vi "Execute Command.vi"(8 "error in (no error)":errorcluster, 9 "Command Name":string, 10 "Robot Actors.lvlib:Command.lvlib:Command.lvclass":refnum<class "Command.lvclass">, 11 "System Actor in":refnum<class "System Actor.lvclass">) -> (0 "error out":errorcluster, 3 "System Actor out":refnum<class "System Actor.lvclass">)   [LabVIEW 2013]
uses:
  <vilib>/ActorFramework/Actor/Actor.lvclass
  System Actor.lvclass
  Command/Command Class/Command.lvclass
  Command/Command Messages/Command Stopped Msg/Command Stopped Msg.lvclass
  Command/Command Messages/Command Started Msg/Command Started Msg.lvclass
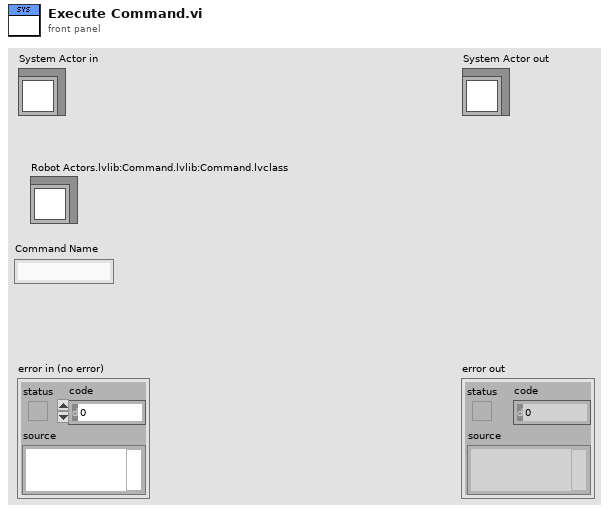
[diagram p1: front panel]
types:
  T1 = typedef "Robot Actors.lvlib/System Actor.lvlib/System Actor.lvclass/System Status.ctl" = cluster{"Instance Name":string, "Command Status":T2, "System Start Time":timestamp, "Next Command ID":dbl}
  T2 = typedef "Robot Actors.lvlib/Command.lvlib/Command.lvclass/Command Status.ctl" = cluster{"Command Name":string, "Command Start Time":timestamp, "Command End Time":timestamp, "Is Command Finished?":bool, "Command ID":dbl, "Command State":T3}
  T3 = typedef "Robot Actors.lvlib/Command.lvlib/Command.lvclass/Command States.ctl" = enum16{"Unknown", "Started", "Stopped", "Finished"}
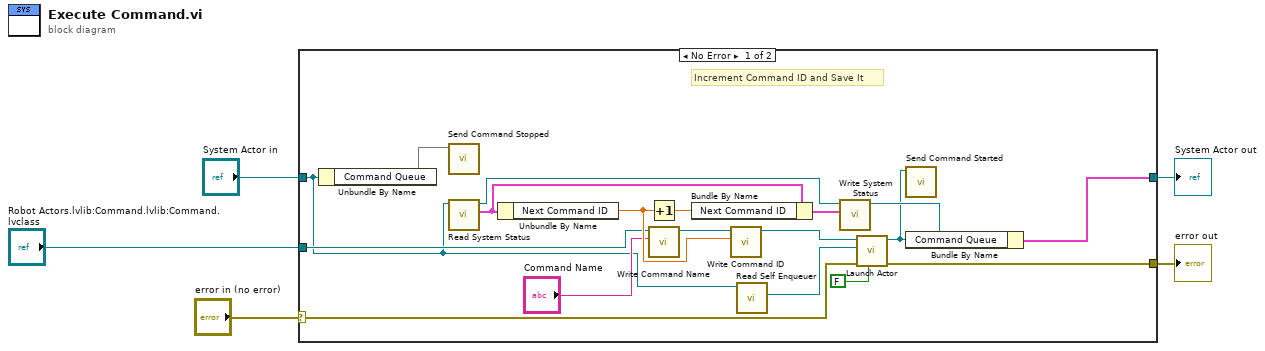
[diagram p0: block diagram]
diagram:
  n1 = case shown="No Error" "error in (no error)" {
    selector: "error in (no error)" -> [w21 w25]
    tunnel: [w22 w25] -> w4
    tunnel: [w20 w24] -> w2
    tunnel: "System Actor in" -> [w7 w24]
    tunnel: "Robot Actors.lvlib:Command.lvlib:Command.lvclass" -> [w10 _]
    frame No Error {
      # "Increment Command ID and Save It"
      n2 = Unbundle By Name(w7) -> ("Command Queue"=w8)
      n3 = call "Send Command Stopped.vi"("Message Enqueuer"=w8) -> ()  [unwired: 9 in, 2 out]
      n4 = call-dynamic "Read System Status.vi"("System Actor in"=w7) -> ("System Status"=w16:T1, "System Actor out"=w18:refnum<class "System Actor.lvclass">)  [unwired: 8 in, 1 out]
      n5 = Unbundle By Name(w16) -> ("Next Command ID"=w14:dbl)
      n6 = Increment(x=w14) -> (x+1=w13:dbl)
      n7 = call-dynamic "Write Command Name.vi"("Command Name"="Command Name", "Command in"=w10) -> ("Command out"=w9:refnum<class "Command.lvclass">)  [unwired: 8 in, 1 out]
      n8 = Bundle By Name(cluster=w16, "Next Command ID"=w13) -> (w15:T1)
      n9 = call-dynamic "Write Command ID.vi"("Command ID"=w14, "Command in"=w9) -> ("Command out"=w19:refnum<class "Command.lvclass">)  [unwired: 8 in, 1 out]
      n10 = call <vilib>:"Read Self Enqueuer.vi"("Actor"=w7) -> ("Self Enqueuer"=w23:refnum<class "Message Enqueuer.lvclass">)  [unwired: 10 in]
      n11 = call-dynamic "Write System Status.vi"("System Status"=w15, "System Actor in"=w18) -> ("System Actor out"=w17:refnum<class "System Actor.lvclass">)  [unwired: 8 in, 1 out]
      n12 = call <vilib>:"Launch Actor.vi"("Open Actor Core front panel? (F)"=FALSE, "error in (no error)"=w21, "Actor-to-Caller Enqueuer"=w23, "Actor"=w19) -> ("error out"=w22:errorcluster, "Caller-To-Actor Enqueuer"=w6:refnum<class "Message Enqueuer.lvclass">)  [unwired: 6 in]
      n13 = call "Send Command Started.vi"("Message Enqueuer"=w6) -> ()  [unwired: 9 in, 2 out]
      n14 = Bundle By Name(cluster=w17, "Command Queue"=w6) -> (w20:cluster{})
    }
    frame Error {
    }
  }
  "error out" <- w4
  "System Actor out" <- w2
